vi "20T_Set_Persistent.vi"(8 "error in (no error)":errorcluster, 10 "20T Control":T1={"Clamp"=TRUE, "Switch Heater"=TRUE, "Go to Zero"=TRUE, "Go to Set"=FALSE, "Go to Hold"=FALSE, "Setpoint (T)"=3.4572, "Rate (T/min)"=0.0, "Set Rate"=FALSE} {"Rate (T/min)" format="%6_5f"; "Setpoint (T)" format="%#4_5f"}, 11 "Mercury Reference In":T2) -> (0 "error out":errorcluster)   [LabVIEW 2019]
uses:
  Equipment/Mercury iXX/Public/Controls/Mercury Reference.ctl
  Equipment/Mercury iXX/Public/Controls/Comms Transport Layer.ctl
  Equipment/Mercury iXX/Private/Controls/Query Dynamic Reference.ctl
  Monitor Communication/Gustav/20T_Control.ctl
  Equipment/Mercury iXX/Public/Libraries/Magnet/Open/Open Magnet Device.vi
  Equipment/Mercury iXX/Public/Libraries/Magnet/Signals/Read/Switch Heater Status (Read).vi
  Equipment/Mercury iXX/Mercury iXX.lvlib
  Equipment/Mercury iXX/Public/Libraries/Magnet.lvlib
panel:
  # "20 T"
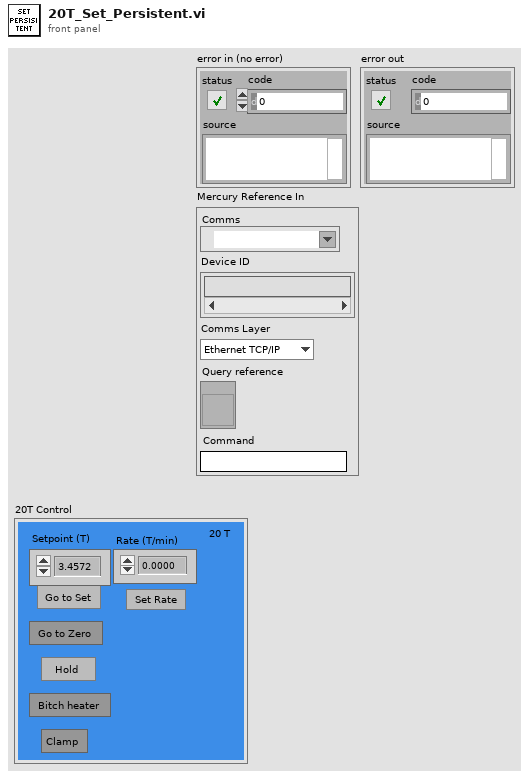
[diagram p1: front panel]
types:
  T1 = typedef "20T_Control.ctl" = cluster{"Clamp":bool, "Switch Heater":bool, "Go to Zero":bool, "Go to Set":bool, "Go to Hold":bool, "Setpoint (T)":dbl, "Rate (T/min)":dbl, "Set Rate":bool}
  T2 = typedef "Mercury iXX.lvlib/Mercury Reference.ctl" = cluster{"Comms":refnum<visa-resource-name>, "Device ID":string[], "Comms Layer":T3, "Command":string, "Query reference":T4}
  T3 = typedef "Mercury iXX.lvlib/Comms Transport Layer.ctl" = enum16{"Ethernet TCP/IP", "USB", "ISOBus - RS-232", "GPIB"}
  T4 = typedef "Mercury iXX.lvlib/Query Dynamic Reference.ctl" = refnum<vi>
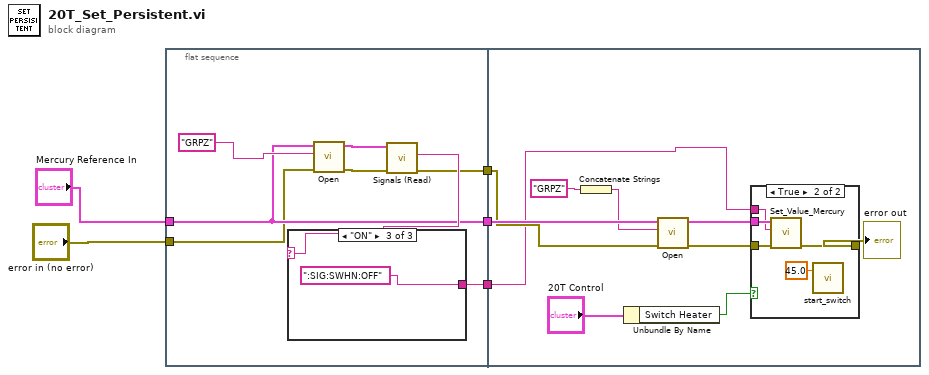
[diagram p0: block diagram]
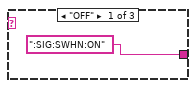
[diagram p2: hidden frame]
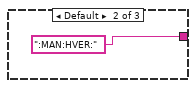
[diagram p3: hidden frame]
diagram:
  n1 = flat-sequence {
    tunnel: "Mercury Reference In" -> [w9]
    tunnel: [w9] -> w4
    tunnel: "error in (no error)" -> [w8]
    tunnel: [w7] -> w2
    tunnel: [w6] -> w1
    tunnel: w4 -> [w26]
    tunnel: w2 -> [w18]
    tunnel: w1 -> [w17]
    frame #0 {
      n2 = call-poly "Open.vi"("error in (no error)"=w8, "Device Identifier"="GRPZ", "Mercury Reference In"=w9) -> ("error out"=w10:errorcluster, "Mercury Reference Out"=w11:T2)  [unwired: 1 in, 6 out]
      n3 = call-poly "Signals (Read).vi"("error in"=w10, "Mercury Reference In"=w11) -> ("error out"=w7:errorcluster, "Switch Heater Status"=w13:string)  [unwired: 6 in, 2 out]
      n4 = case shown="\"ON\"" w13 {
        tunnel: [":SIG:SWHN:ON" ":MAN:HVER:" ":SIG:SWHN:OFF"] -> w6
        frame "OFF" {
        }
        frame Default {
        }
        frame "ON" {
        }
      }
    }
    frame #1 {
      n5 = Concatenate Strings("GRPZ" ("Device Identifier")) -> (w23:string)
      n6 = Unbundle By Name("20T Control") -> ("Switch Heater"=w19:bool)
      n7 = call-poly "Open.vi"("error in (no error)"=w18, "Device Identifier"=w23, "Mercury Reference In"=w26) -> ("error out"=w24:errorcluster, "Mercury Reference Out"=w25:T2)  [unwired: 1 in, 6 out]
      n8 = case shown="True" w19 {
        tunnel: w25 -> [_ w32]
        tunnel: w24 -> [w27 w29]
        tunnel: [w27 w30] -> w22
        tunnel: w17 -> [_ w31]
        frame False {
        }
        frame True {
          n9 = call "Set_Value_Mercury.vi"("error in"=w29, "Noun(s)"=w31, "Mercury Reference In"=w32) -> ("error out"=w30:errorcluster)  [unwired: 7 in, 1 out]
          n10 = call "start_switch.vi"("Switch heater time"=45.0) -> ()  [unwired: 2 in]
        }
      }
      "error out" <- w22
    }
  }
